vi "Scale Arbitrary Waveform.vi"(8 "error in (no error)":errorcluster, 10 "Arbitrary Waveform Data":dbl[](array[numeric]), 11 "VISA resource name":refnum<visa-resource-name>) -> (0 "error out":errorcluster, 2 "Scaled Arbitrary Waveform Data":i16[](array[numeric]), 3 "VISA resource name out":refnum<visa-resource-name>)   [LabVIEW 2020, in "Agilent 33XXX Series.lvlib"]
doc: "This VI scales a data array so that the maximum (positive or negative) value in the array corresponds to the maximum allowed value (positive or negative) for the instrument.\n\n33120a: -2047 to 2047\n33220a/33250a: -8191 to 8191"
uses:
  Agilent 33XXX Series.lvlib
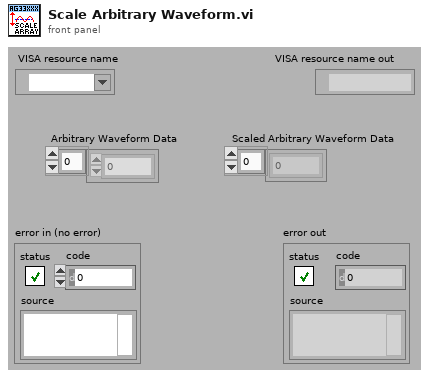
[diagram p1: front panel]
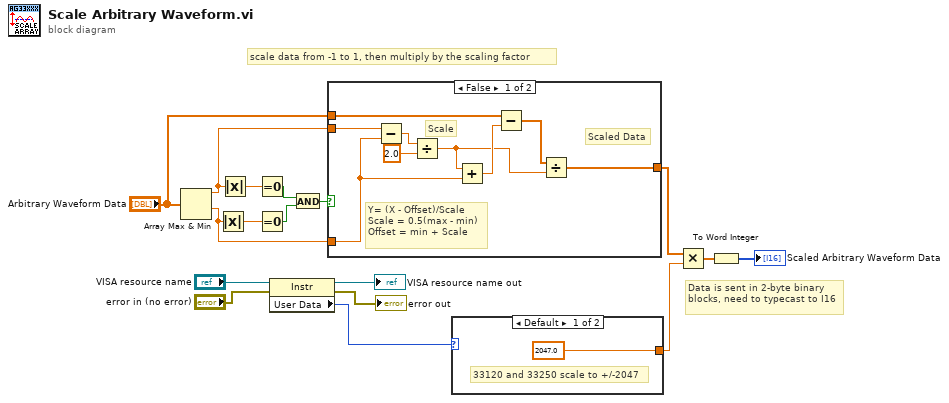
[diagram p0: block diagram]
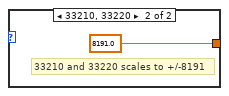
[diagram p2: hidden frame]
diagram:
  # "Data is sent in 2-byte binary blocks, need to typecast to I16"
  # "scale data from -1 to 1, then multiply by the scaling factor"
  n1 = Array Max & Min(array="Arbitrary Waveform Data") -> (max value=w3:dbl, min value=w1:dbl)  [unwired: 2 out]
  n2 = Absolute Value(x=w1) -> (abs(x)=w13:dbl)
  n3 = Absolute Value(x=w3) -> (abs(x)=w12:dbl)
  n4 = Equal To 0?(x=w12) -> (x = 0?=w15:bool)
  n5 = Equal To 0?(x=w13) -> (x = 0?=w14:bool)
  n6 = property class="Instr"(reference="VISA resource name", error in="error in (no error)") -> (reference out=→"VISA resource name out":refnum<visa-resource-name>, error out=→"error out":errorcluster, "User Data"=w5:u32)
  n7 = And(x=w15, y=w14) -> (x .and. y?=w11:bool)
  n8 = case shown="False" w11 {
    tunnel: w3 -> [w26 _]
    tunnel: "Arbitrary Waveform Data" -> [w23 w27]
    tunnel: [w19 w27] -> w10
    tunnel: w1 -> [w18 _]
    frame False {
      # "Y= (X - Offset)/Scale\nScale = 0.5(max - min)\nOffset = min + Scale"
      # "Scale"
      # "Scaled Data"
      n9 = Subtract(x=w26, y=w18) -> (x-y=w25:dbl)
      n10 = Divide(x=w25, y=2.0) -> (x/y=w20:dbl)
      n11 = Add(x=w20, y=w18) -> (x+y=w22:dbl)
      n12 = Subtract(x=w23, y=w22) -> (x-y=w21:dbl[])
      n13 = Divide(x=w21, y=w20) -> (x/y=w19:dbl[])
    }
    frame True {
      # "This case occurs when all the data in the table\nare zeros, thus, the maximum and the minimum\nare the same and no division required."
    }
  }
  n14 = case shown="Default" w5 {
    tunnel: [2047.0 ("y") 8191.0 ("y")] -> w4
    frame Default {
      # "33120 and 33250 scale to +/-2047"
    }
    frame 33210, 33220 {
      # "33210 and 33220 scales to +/-8191"
    }
  }
  n15 = Multiply(x=w10, y=w4) -> (x*y=w16:dbl[])
  n16 = To Word Integer(number=w16) -> (16bit integer=→"Scaled Arbitrary Waveform Data":i16[])
